vi "MGCF_main.vi"() -> ()   [LabVIEW 2015]
uses:
  Classes/System/System.lvclass/System.ctl
  Classes/AssetInterface/Interface_Asset.lvclass
  Classes/DispatchInterface/Interface_Dispatch.lvclass
  Classes/System/System.lvclass
panel:
  in  "stop":bool
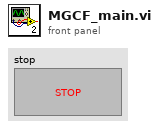
[diagram p1: front panel]
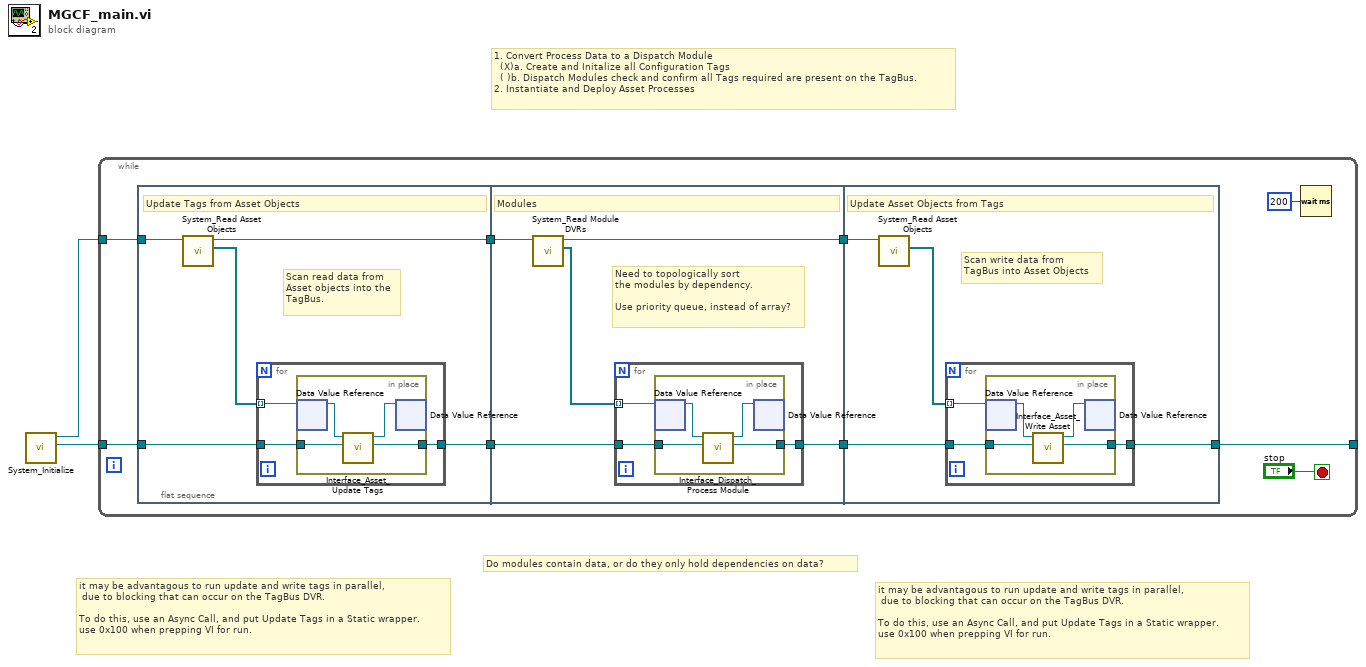
[diagram p0: block diagram]
diagram:
  # "Do modules contain data, or do they only hold dependencies on data?"
  # "it may be advantagous to run update and write tags in parallel,\n due to blocking that can occur on the TagBus DVR.\n\nTo do this, use an Async Call, and put Update Tags in a Static wrapper.\nuse 0x100 when prepping VI for run."
  # "it may be advantagous to run update and write tags in parallel,\n due to blocking that can occur on the TagBus DVR.\n\nTo do this, use an Async Call, and put Update Tags in a Static wrapper.\nuse 0x100 when prepping VI for run."
  # "1. Convert Process Data to a Dispatch Module\n  (X)a. Create and Initalize all Configuration Tags\n  ( )b. Dispatch Modules check and confirm all Tags required are present on the TagBus.\n2. Instantiate and Deploy Asset Processes"
  n1 = call "System_Initialize.vi"() -> ("TagBus DVR"=w1:refnum<data-value>, "System DVR out"=w2:refnum<data-value>)  [unwired: 10 in]
  n2 = while {
    tunnel: w1 -> [w7]
    tunnel: w2 -> [w9]
    tunnel: [w8] -> _
    stop <- "stop" stop-if-true
    n3 = flat-sequence {
      tunnel: w9 -> [w16]
      tunnel: [w14] -> w6
      tunnel: w7 -> [w13]
      tunnel: [w12] -> w5
      tunnel: w6 -> [w28]
      tunnel: [w27] -> w4
      tunnel: w5 -> [w25]
      tunnel: [w24] -> w3
      tunnel: [w37] -> w8
      tunnel: w4 -> [w39]
      tunnel: w3 -> [w36]
      frame #0 {
        # "Scan read data from\nAsset objects into the\nTagBus."
        # "Update Tags from Asset Objects"
        n4 = call "System_Read Asset Objects.vi"("data value reference"=w16) -> ("Asset DVR Array"=w15:refnum<data-value>[], "data value reference out"=w14:refnum<data-value>)  [unwired: 9 in]
        n5 = for {
          tunnel: w15 -> [w17] mode=indexing
          tunnel: w13 -> [w19]
          tunnel: [w18] -> w12
          n6 = in-place {
            in-place-border: w19 -> [w23]
            in-place-border: [w22] -> w18
            n7 = in-place-dvr #1(w17) -> (w21:refnum<class "Interface_Asset.lvclass">)  [unwired: 1 out]
            n8 = call-dynamic "Interface_Asset_Update Tags.vi"("TagBus DVR"=w23, "Asset_Interface in"=w21) -> ("TagBus DVR out"=w22:refnum<data-value>, "Asset_Interface out"=w20:refnum<class "Interface_Asset.lvclass">)  [unwired: 7 in, 1 out]
            n9 = in-place-dvr #1(w20) -> ()  [unwired: 2 out]
          }
        }
      }
      frame #1 {
        # "Need to topologically sort\nthe modules by dependency.\n\nUse priority queue, instead of array?"
        # "Modules"
        n10 = call "System_Read Module DVRs.vi"("Data Value Reference in"=w28) -> ("Dispatch Module DVR Array"=w26:refnum<data-value>[], "Data Value Reference out"=w27:refnum<data-value>)  [unwired: 9 in]
        n11 = for {
          tunnel: w26 -> [w29] mode=indexing
          tunnel: w25 -> [w31]
          tunnel: [w30] -> w24
          n12 = in-place {
            in-place-border: w31 -> [w33]
            in-place-border: [w32] -> w30
            n13 = in-place-dvr #2(w29) -> (w35:refnum<class "Interface_Dispatch.lvclass">)  [unwired: 1 out]
            n14 = call-dynamic "Interface_Dispatch_Process Module.vi"("TagBus DVR"=w33, "Interface_Dispatch in"=w35) -> ("TagBus DVR out"=w32:refnum<data-value>, "Interface_Dispatch out"=w34:refnum<class "Interface_Dispatch.lvclass">)  [unwired: 7 in, 1 out]
            n15 = in-place-dvr #2(w34) -> ()  [unwired: 2 out]
          }
        }
      }
      frame #2 {
        # "Scan write data from\nTagBus into Asset Objects"
        # "Update Asset Objects from Tags"
        n16 = call "System_Read Asset Objects.vi"("data value reference"=w39) -> ("Asset DVR Array"=w38:refnum<data-value>[])  [unwired: 9 in, 1 out]
        n17 = for {
          tunnel: w38 -> [w40] mode=indexing
          tunnel: w36 -> [w42]
          tunnel: [w41] -> w37
          n18 = in-place {
            in-place-border: w42 -> [w44]
            in-place-border: [w43] -> w41
            n19 = in-place-dvr #3(w40) -> (w45:refnum<class "Interface_Asset.lvclass">)  [unwired: 1 out]
            n20 = call-dynamic "Interface_Asset_Write Asset.vi"("TagBus DVR"=w44, "Asset_Interface in"=w45) -> ("TagBus DVR out"=w43:refnum<data-value>, "Asset_Interface out"=w46:refnum<class "Interface_Asset.lvclass">)  [unwired: 7 in, 1 out]
            n21 = in-place-dvr #3(w46) -> ()  [unwired: 2 out]
          }
        }
      }
    }
    n22 = Wait (ms)(milliseconds to wait=u32 200) -> ()  [unwired: 1 out]
  }
